vi "ElevatorStateSelect.vi"() -> (2 "Elevator State":string)   [LabVIEW 2018]
uses:
  Inputs_DriverStation.vi
  RobotStates.vi
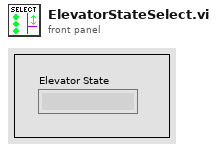
[diagram p1: front panel]
types:
  T1 = cluster{"Elevator_Stow":bool, "Cargo_Ground":bool, "Cargo_Feeder":bool, "Cargo_Ship":bool, "Cargo_Rocket_1":bool, "Cargo_Rocket_2":bool, "Cargo_Rocket_3":bool, "Hatch_Ground":bool, "Hatch_Feeder":bool, "Hatch_Ship":bool, "Hatch_Rocket_1":bool, "Hatch_Rocket_2":bool, "Hatch_Rocket_3":bool, "Climb":bool}
  T2 = cluster{"Trigger":bool, "Trigger":bool, "Trigger":bool, "Trigger":bool, "Trigger":bool, "Trigger":bool, "Trigger":bool, "Trigger":bool, "Trigger":bool, "Trigger":bool, "Trigger":bool, "Trigger":bool, "Trigger":bool, "Trigger":bool}
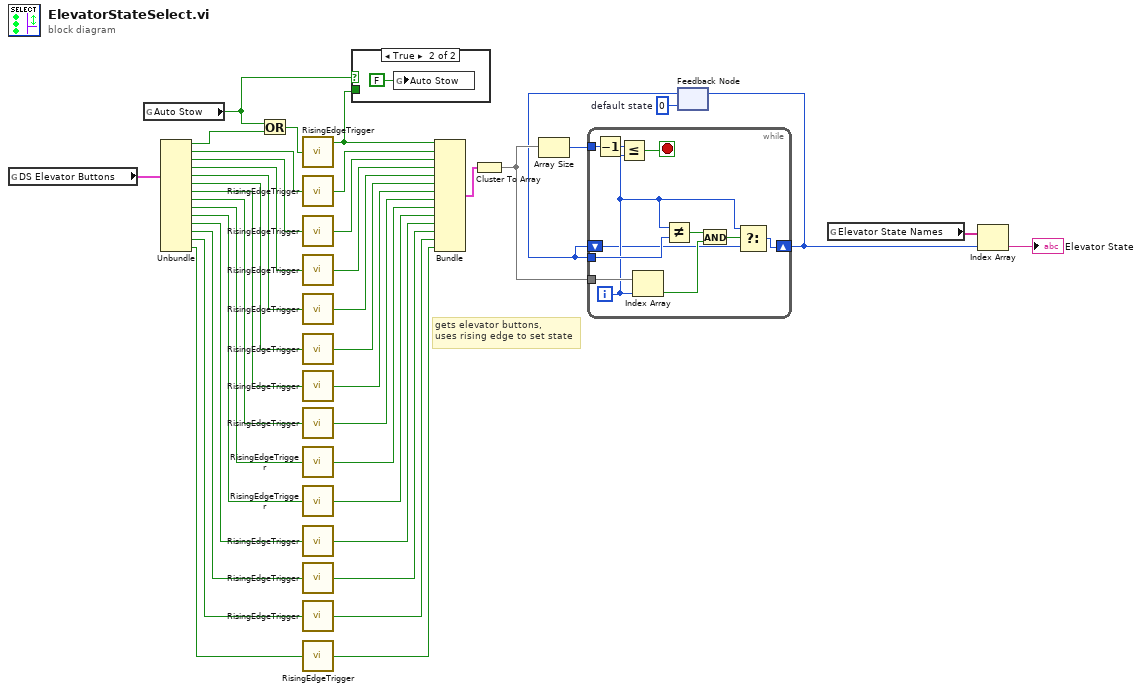
[diagram p0: block diagram]
diagram:
  w38 = 0  # default state
  # "gets elevator buttons,\nuses rising edge to set state"
  n1 = global read "Inputs_DriverStation.vi" "DS Elevator Buttons"() -> (w32:T1)
  n2 = global read "RobotStates.vi" "Auto Stow"() -> (w2:bool)
  n3 = Unbundle(w32) -> ("Elevator_Stow"=w3:bool, "Cargo_Ground"=w34:bool, "Cargo_Feeder"=w33:bool, "Cargo_Ship"=w28:bool, "Cargo_Rocket_1"=w27:bool, "Cargo_Rocket_2"=w26:bool, "Cargo_Rocket_3"=w25:bool, "Hatch_Ground"=w20:bool, "Hatch_Feeder"=w19:bool, "Hatch_Ship"=w18:bool, "Hatch_Rocket_1"=w17:bool, "Hatch_Rocket_2"=w16:bool, "Hatch_Rocket_3"=w15:bool, "Climb"=w6:bool)
  n4 = Or(x=w2, y=w3) -> (x .or. y?=w4:bool)
  n5 = call "RisingEdgeTrigger.vi"("Raw Signal"=w4) -> ("Trigger"=w1:bool)
  n6 = call "RisingEdgeTrigger.vi"("Raw Signal"=w34) -> ("Trigger"=w36:bool)
  n7 = call "RisingEdgeTrigger.vi"("Raw Signal"=w33) -> ("Trigger"=w35:bool)
  n8 = call "RisingEdgeTrigger.vi"("Raw Signal"=w28) -> ("Trigger"=w24:bool)
  n9 = call "RisingEdgeTrigger.vi"("Raw Signal"=w27) -> ("Trigger"=w23:bool)
  n10 = call "RisingEdgeTrigger.vi"("Raw Signal"=w26) -> ("Trigger"=w22:bool)
  n11 = call "RisingEdgeTrigger.vi"("Raw Signal"=w25) -> ("Trigger"=w21:bool)
  n12 = call "RisingEdgeTrigger.vi"("Raw Signal"=w20) -> ("Trigger"=w14:bool)
  n13 = call "RisingEdgeTrigger.vi"("Raw Signal"=w19) -> ("Trigger"=w13:bool)
  n14 = call "RisingEdgeTrigger.vi"("Raw Signal"=w18) -> ("Trigger"=w12:bool)
  n15 = call "RisingEdgeTrigger.vi"("Raw Signal"=w17) -> ("Trigger"=w11:bool)
  n16 = call "RisingEdgeTrigger.vi"("Raw Signal"=w16) -> ("Trigger"=w10:bool)
  n17 = call "RisingEdgeTrigger.vi"("Raw Signal"=w15) -> ("Trigger"=w9:bool)
  n18 = call "RisingEdgeTrigger.vi"("Raw Signal"=w6) -> ("Trigger"=w5:bool)
  n19 = case shown="True" w2 {
    tunnel: w1 -> [_ _]
    frame False {
    }
    frame True {
      n20 = global write "RobotStates.vi" "Auto Stow"(FALSE ("Auto Stow")) -> ()
    }
  }
  n21 = Bundle("Trigger"=w1, "Trigger"=w36, "Trigger"=w35, "Trigger"=w24, "Trigger"=w23, "Trigger"=w22, "Trigger"=w21, "Trigger"=w14, "Trigger"=w13, "Trigger"=w12, "Trigger"=w11, "Trigger"=w10, "Trigger"=w9, "Trigger"=w5) -> (w8:T2)  [unwired: 1 in]
  n22 = Cluster To Array(cluster=w8) -> (array=w39:bool[])
  n23 = Array Size(array=w39) -> (size(s)=w7:i32)
  n24 = feedback #1(w38) -> (w37:i32)
  n25 = while {
    tunnel: w39 -> [w51]
    tunnel: w37 -> [w46]
    tunnel: w7 -> [w44]
    shift-right: [w47] -> w30
    shift-left: w37 -> [w41]
    i -> [w45]
    stop <- w43 stop-if-true
    n26 = Decrement(x=w44) -> (x-1=w42:i32)
    n27 = Less Or Equal?(x=w42, y=w45) -> (x <= y?=w43:bool)
    n28 = Index Array(array=w51, index=w45) -> (element=w49:bool)
    n29 = Not Equal?(x=w45, y=w46) -> (x != y?=w48:bool)
    n30 = And(x=w48, y=w49) -> (x .and. y?=w50:bool)
    n31 = Select(t=w45, s=w50, f=w41) -> (s? t:f=w47:i32)
  }
  n32 = feedback-in #1(w30) -> ()
  n33 = global read "RobotStates.vi" "Elevator State Names"() -> (w31:string[])
  n34 = Index Array(array=w31, index=w30) -> (element=→"Elevator State":string)
